vi "Get Bytes.vi"(11 "MsgPackMap in":refnum<class "MsgPackMap.lvclass">) -> (2 "Array":u8[](array[numeric]), 3 "MsgPackMap out":refnum<class "MsgPackMap.lvclass">)   [LabVIEW 2020, in "wamplv.lvlib" / "MsgPackMap.lvclass"]
uses:
  MsgPackMap.lvclass
  MsgPackMap.lvclass/MsgPackMap.ctl
  Format bytes.ctl
  MessagePack.lvclass
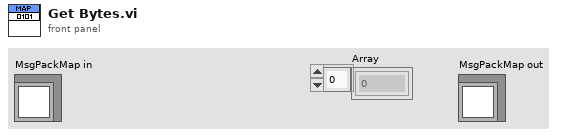
[diagram p1: front panel]
types:
  T1 = typedef "wamplv.lvlib/MessagePack.lvclass/Format bytes.ctl" = u8
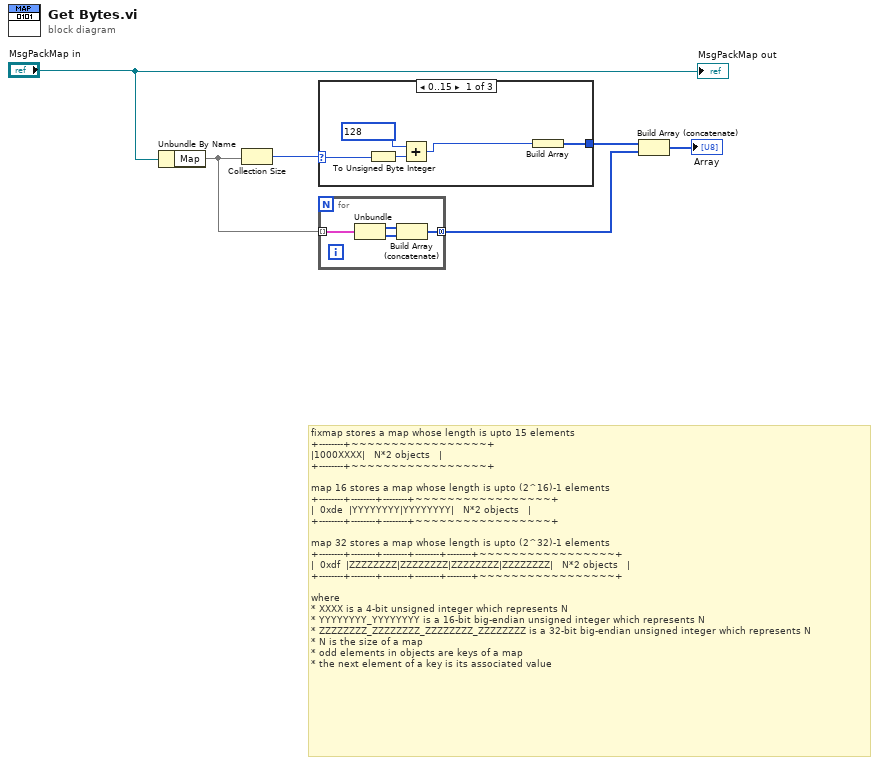
[diagram p0: block diagram]
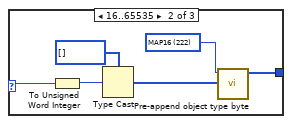
[diagram p2: hidden frame]
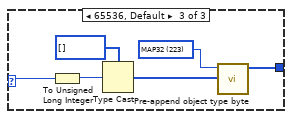
[diagram p3: hidden frame]
diagram:
  # "fixmap stores a map whose length is upto 15 elements\n+--------+~~~~~~~~~~~~~~~~~+\n|1000XXXX|   N*2 objects   |\n+--------+~~~~~~~~~~~~~~~~~+\n\nmap 16 stores a map whose length is upto (2^16)-1 elements\n+--------+--------+--------+~~~~~~~~~~~~~~~~~+\n|  0xde  |YYYYYYYY|YYYYYYYY|   N*2 objects   |\n+--------+--------+--------+~~~~~~~~~~~~~~~~~+\n\nmap 32 stores a map whose length is upto (2^32)-1 elements\n+--------+--------+--------+--------+--------+~~~~~~~~~~~~~~~~~+\n|  0xdf  |ZZZZZZZZ|ZZZZZZZZ|ZZZZZZZZ|ZZZZZZZZ|   N*2 objects   |\n+--------+--------+--------+--------+--------+~~~~~~~~~~~~~~~~~+\n\nwhere\n* XXXX is a 4-bit unsigned integer which represents N\n* YYYYYYYY_YYYYYYYY is a 16-bit big-endian unsigned integer which represents N\n* ZZZZZZZZ_ZZZZZZZZ_ZZZZZZZZ_ZZZZZZZZ is a 32-bit big-endian unsigned integer which represents N\n* N is the size of a map\n* odd elements in objects are keys of a map\n* the next element of a key is its associated value"
  n1 = Unbundle By Name("MsgPackMap in") -> ("Map"=w3:map{u8[], u8[]})
  n2 = Collection Size(1:w3) -> (0:w2:i32)
  n3 = case shown="0..15" w2 {
    selector: w2 -> [w10 w17 w23]
    tunnel: [w8 w13 w19] -> w6
    frame 0..15 {
      n4 = To Unsigned Byte Integer(number=w10) -> (unsigned 8bit integer=w9:u8)
      n5 = Add(x=u8 128 ("y"), y=w9) -> (x+y=w7:u8)
      n6 = Build Array(w7) -> (w8:u8[])
    }
    frame 16..65535 {
      w12 = T1 222 items=["nil"=192, "UINT8"=204, "UINT16"=205, "UINT32"=206, "UINT64"=207, "INT8"=208, "INT16"=209, "INT32"=210, "INT64"=211, "FALSE"=194, "TRUE"=195, "SGL"=202, "DBL"=203, "ARRAY16"=220, "ARRAY32"=221, "MAP16"=222, "MAP32"=223] ("Format byte")
      n7 = To Unsigned Word Integer(number=w17) -> (unsigned 16bit integer=w15:u16)
      n8 = Type Cast(type=u8[] [] ("bytes"), x=w15) -> (*(type *) &x=w14:u8[])
      n9 = call "Pre-append object type byte.vi"("data in"=w14, "Format byte"=w12) -> ("bytes add"=w13:u8[])  [unwired: 9 in]
    }
    frame 65536, Default {
      w18 = T1 223 items=["nil"=192, "UINT8"=204, "UINT16"=205, "UINT32"=206, "UINT64"=207, "INT8"=208, "INT16"=209, "INT32"=210, "INT64"=211, "FALSE"=194, "TRUE"=195, "SGL"=202, "DBL"=203, "ARRAY16"=220, "ARRAY32"=221, "MAP16"=222, "MAP32"=223] ("Format byte")
      n10 = To Unsigned Long Integer(number=w23) -> (unsigned 32bit integer=w21:u32)
      n11 = Type Cast(type=u8[] [] ("bytes"), x=w21) -> (*(type *) &x=w20:u8[])
      n12 = call "Pre-append object type byte.vi"("data in"=w20, "Format byte"=w18) -> ("bytes add"=w19:u8[])  [unwired: 9 in]
    }
  }
  n13 = for {
    tunnel: w3 -> [w27] mode=indexing
    tunnel: [w24] -> w1 mode=concatenating
    n14 = Unbundle(w27) -> ("Key"=w26:u8[], "Value"=w25:u8[])
    n15 = Build Array (concatenate)(w26, w25) -> (w24:u8[])
  }
  n16 = Build Array (concatenate)(w6, w1) -> (→"Array":u8[])
  "MsgPackMap out" <- "MsgPackMap in"
